vi "DropCarryOffset.vi"(9 "Lights Values":T1=[[{"Port"=1, "On Value"=255, "Off Value"=255}, {"Port"=2, "On Value"=0, "Off Value"=0}, {"Port"=3, "On Value"=0, "Off Value"=0}], [{"Port"=4, "On Value"=0, "Off Value"=0}, {"Port"=5, "On Value"=0, "Off Value"=0}, {"Port"=6, "On Value"=0, "Off Value"=0}], [{"Port"=7, "On Value"=0, "Off Value"=0}, {"Port"=8, "On Value"=0, "Off Value"=0}, {"Port"=9, "On Value"=0, "Off Value"=0}], [{"Port"=10, "On Value"=0, "Off Value"=0}, {"Port"=11, "On Value"=0, "Off Value"=0}, {"Port"=12, "On Value"=0, "Off Value"=0}], [{"Port"=13, "On Value"=0, "Off Value"=0}, {"Port"=14, "On Value"=0, "Off Value"=0}, {"Port"=15, "On Value"=0, "Off Value"=0}], [{"Port"=58, "On Value"=255, "Off Value"=0}, {"Port"=0, "On Value"=0, "Off Value"=0}, {"Port"=0, "On Value"=0, "Off Value"=0}], [{"Port"=49, "On Value"=255, "Off Value"=0}, {"Port"=0, "On Value"=0, "Off Value"=0}, {"Port"=0, "On Value"=0, "Off Value"=0}], [{"Port"=52, "On Value"=255, "Off Value"=0}, {"Port"=0, "On Value"=0, "Off Value"=0}, {"Port"=0, "On Value"=0, "Off Value"=0}], [{"Port"=55, "On Value"=255, "Off Value"=0}, {"Port"=0, "On Value"=0, "Off Value"=0}, {"Port"=0, "On Value"=0, "Off Value"=0}], [{"Port"=46, "On Value"=255, "Off Value"=0}, {"Port"=0, "On Value"=0, "Off Value"=0}, {"Port"=0, "On Value"=0, "Off Value"=0}], [{"Port"=61, "On Value"=0, "Off Value"=0}, {"Port"=0, "On Value"=0, "Off Value"=0}, {"Port"=0, "On Value"=0, "Off Value"=0}]], 10 "Buttons":bool[](array[boolean]), 11 "Presets":T2) -> (2 "container?":bool)   [LabVIEW 2014]
doc: "If the container/tote button is pressed, change value to 0 or offset and turn light on if the new value is the container offset"
uses:
  PresetValues.ctl
  LEDdriver/LEDPorts.ctl
  <vilib>/Rock Robotics/Network Tables/SD Read Number.vi
  <vilib>/Rock Robotics/Network Tables/SD Write Boolean.vi
  <vilib>/Rock Robotics/Network Tables/SD Write Number.vi
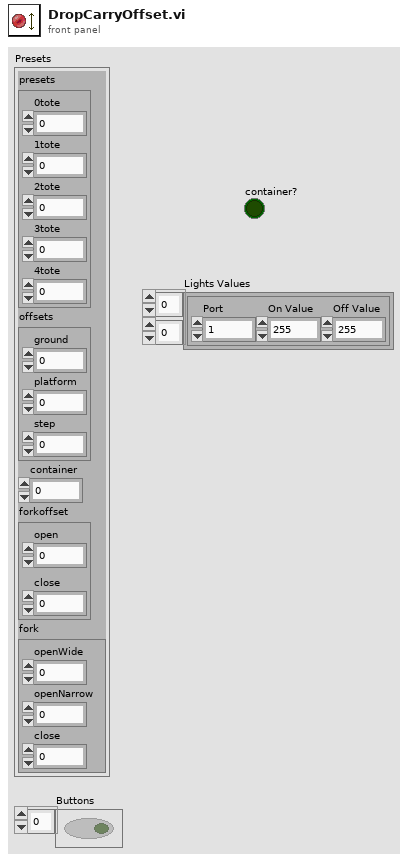
[diagram p1: front panel]
types:
  T1 = typedef "LEDPorts.ctl" = cluster{"Port":i16, "On Value":u8, "Off Value":u8}[][]
  T2 = typedef "PresetValues.ctl" = cluster{"presets":cluster{"0tote":dbl, "1tote":dbl, "2tote":dbl, "3tote":dbl, "4tote":dbl}, "offsets":cluster{"ground":dbl, "platform":dbl, "step":dbl}, "container":dbl, "forkoffset":cluster{"open":dbl, "close":dbl}, "fork":cluster{"openWide":dbl, "openNarrow":dbl, "close":dbl}}
  T3 = cluster{"Port":i16, "On Value":u8, "Off Value":u8}[]
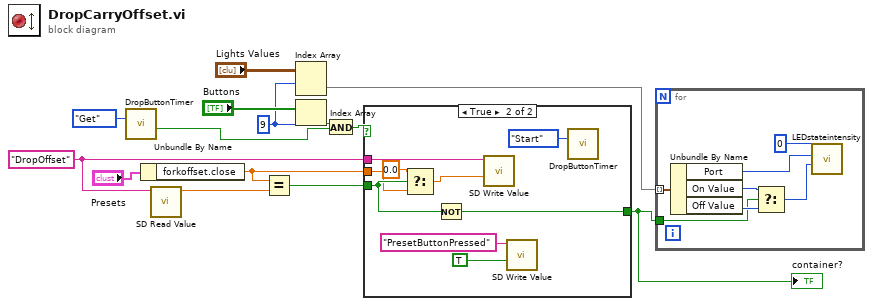
[diagram p0: block diagram]
diagram:
  w11 = "DropOffset" ("Name")
  w7 = 9 ("index")
  n1 = call "DropButtonTimer.vi"("action"=enum16{"Get", "Start"}."Get") -> ("Time elapsed"=w1:bool)  [unwired: 10 in]
  n2 = Unbundle By Name("Presets") -> ("forkoffset.close"=w10:dbl)
  n3 = call-poly <vilib>:"SD Read Value.vi"("Name"=w11) -> ("Numeric"=w9:dbl)  [unwired: 8 in, 2 out]
  n4 = Equal?(x=w10, y=w9) -> (x = y?=w3:bool)
  n5 = Index Array(array="Lights Values", index (row)=w7) -> (element=w6:T3)  [unwired: 1 in]
  n6 = Index Array(array="Buttons", index=w7) -> (element=w14:bool)
  n7 = And(x=w14, y=w1) -> (x .and. y?=w2:bool)
  n8 = case shown="True" w2 {
    tunnel: w10 -> [_ w19]
    tunnel: w11 -> [_ w23]
    tunnel: w3 -> [w15 w22]
    tunnel: [w15 w21] -> w5
    frame False {
    }
    frame True {
      n9 = Select(t=0.0 ("f"), s=w22, f=w19) -> (s? t:f=w24:dbl)
      n10 = Not(x=w22) -> (.not. x?=w21:bool)
      n11 = call-poly <vilib>:"SD Write Value.vi"("Numeric"=w24, "Name"=w23) -> ()  [unwired: 8 in, 2 out]
      n12 = call-poly <vilib>:"SD Write Value.vi"("Boolean"=TRUE, "Name"="PresetButtonPressed") -> ()  [unwired: 8 in, 2 out]
      n13 = call "DropButtonTimer.vi"("action"=enum16{"Get", "Start"}."Start") -> ()  [unwired: 10 in, 1 out]
    }
  }
  "container?" <- w5
  n14 = for {
    tunnel: w6 -> [w31] mode=indexing
    tunnel: w5 -> [w25]
    n15 = Unbundle By Name(w31) -> ("Port"=w29:i16, "On Value"=w28:u8, "Off Value"=w27:u8)
    n16 = Select(t=w28, s=w25, f=w27) -> (s? t:f=w26:u8)
    n17 = call "LEDstateintensity.vi"("intensity"=w26, "port"=w29, "Id"=i16 0) -> ()  [unwired: 6 in, 3 out]
  }
